vi "Quadrature Encoder.vi"() -> ()   [LabVIEW 2010]
uses:
  <vilib>/DAQmx/read.llb/DAQmx Read (Counter DBL 1Chan 1Samp).vi
  <vilib>/DAQmx/create/channels.llb/DAQmx Create Channel (CI-Count Edges).vi
  <vilib>/daqmx/miscellaneous.llb/DAQmx Fill In Error Info.vi
panel:
  out "Position":dbl format="%0.2f"
  in  "stop":bool
  in  "counter":tag
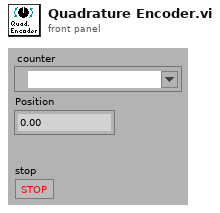
[diagram p1: front panel]
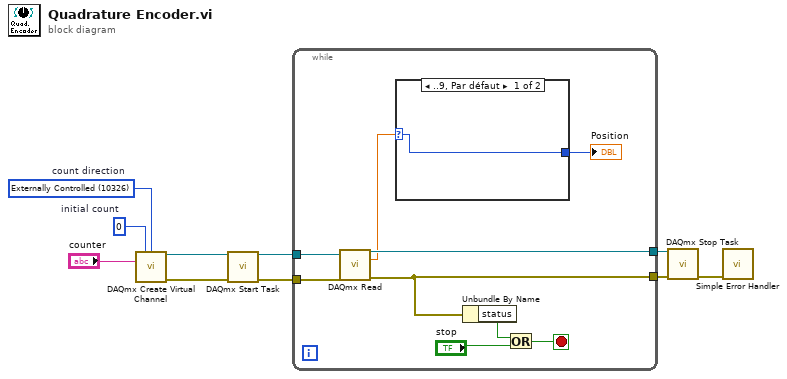
[diagram p0: block diagram]
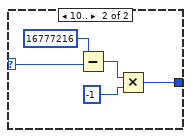
[diagram p2: hidden frame]
diagram:
  w1 = 0  # initial count
  w5 = 10326 items=["Count Up"=10128, "Count Down"=10124, "Externally Controlled"=10326]  # count direction
  n1 = call-poly <vilib>:"DAQmx Create Virtual Channel.vi"("initial count"=w1, "count direction"=w5, "counter"="counter") -> ("task out"=w4:refnum<k21>, "error out"=w3:errorcluster)  [unwired: 11 in]
  n2 = call <vilib>:"DAQmx Start Task.vi"("task/channels in"=w4, "error in"=w3) -> ("task out"=w9:refnum<k21>, "error out"=w8:errorcluster)  [unwired: 12 in]
  n3 = while {
    tunnel: w9 -> [w19]
    tunnel: w8 -> [w14]
    tunnel: [w18] -> w7
    tunnel: [w13] -> w2
    stop <- w16 stop-if-true
    n4 = call-poly <vilib>:"DAQmx Read.vi"("task/channels in"=w19, "error in"=w14) -> ("task out"=w18:refnum<k21>, "data"=w12:dbl, "error out"=w13:errorcluster)  [unwired: 11 in]
    n5 = case shown="..9, Par défaut" w12 {
      selector: w12 -> [w20 w24]
      tunnel: [w20 w21] -> w11
      frame ..9, Default {
      }
      frame 10.. {
        n6 = Subtract(x=16777216, y=w24) -> (x-y=w23:i32)
        n7 = Multiply(x=w23, y=-1) -> (x*y=w21:i32)
      }
    }
    "Position" <- w11
    n8 = Unbundle By Name(w13) -> ("status"=w17:bool)
    n9 = Or(x=w17, y="stop") -> (x .or. y?=w16:bool)
  }
  n10 = call <vilib>:"DAQmx Stop Task.vi"("task/channels in"=w7, "error in"=w2) -> ("error out"=w6:errorcluster)  [unwired: 12 in, 1 out]
  n11 = call <vilib>:"Simple Error Handler.vi"("error in (no error)"=w6) -> ()  [unwired: 4 in, 5 out]
